vi "Read PIDs from Config.vi"(8 "error in (no error)":errorcluster, 10 "keys":string[](array[string]), 11 "Settings":variant) -> (0 "error out":errorcluster, 2 "Array":T1[](array[typedef]), 3 "Settings out":variant)   [LabVIEW 2019, in "DriveOld.lvlib" / "Drive.lvclass"]
doc: "This VI reads the PIDF values from the configuration file and returns an array of the PIDF's requested from the specific variant."
uses:
  Drive.lvclass
  <vilib>/Rock Robotics/WPI/ThirdParty/Phoenix-LabVIEW/Motor Controller/Controls/CTRE_Phoenix_MotorControl_SlotStructure.ctl
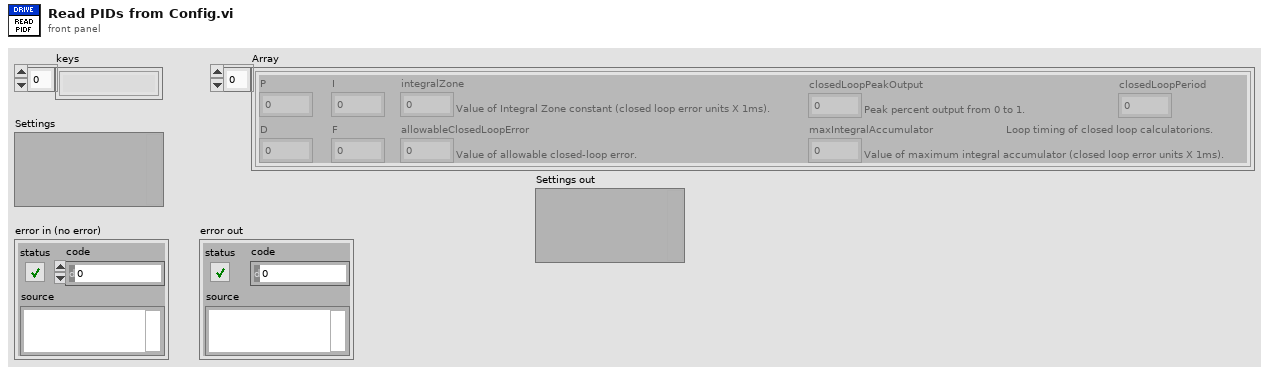
[diagram p1: front panel]
types:
  T1 = typedef "CTRE_Phoenix_MotorControl_SlotStructure.ctl" = cluster{"P":dbl, "I":dbl, "D":dbl, "F":dbl, "integralZone":dbl, "allowableClosedLoopError":i32, "maxIntegralAccumulator":dbl, "closedLoopPeakOutput":dbl, "closedLoopPeriod":i32}
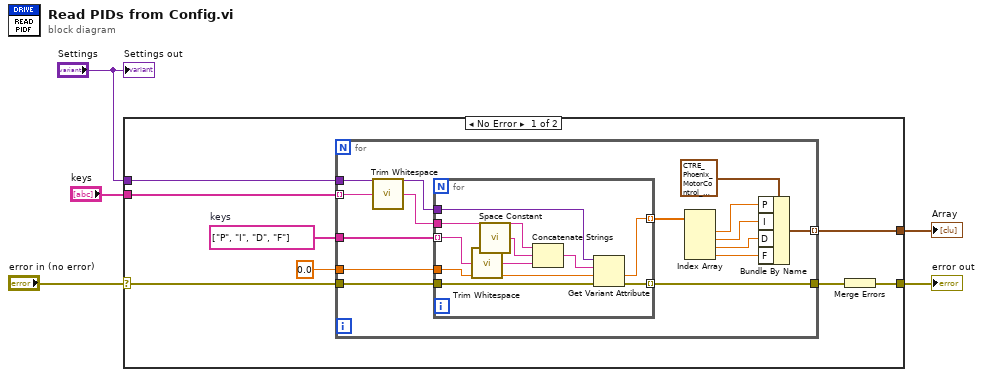
[diagram p0: block diagram]
diagram:
  n1 = case shown="No Error" "error in (no error)" {
    selector: "error in (no error)" -> [w10 w38]
    tunnel: [w12 w38] -> w5
    tunnel: "keys" -> [w9 _]
    tunnel: "Settings" -> [w8 _]
    tunnel: [w6 _] -> w1
    frame No Error {
      w7 = string[] ["P", "I", "D", "F"]  # keys
      n2 = for {
        tunnel: w8 -> [w27]
        tunnel: w9 -> [w22] mode=indexing
        tunnel: w10 -> [w26]
        tunnel: [w25] -> w11
        tunnel: 0.0 -> [w24]
        tunnel: w7 -> [w23]
        tunnel: [w15] -> w6 mode=indexing
        n3 = call <vilib>:"Trim Whitespace.vi"("string"=w22) -> ("trimmed string"=w21:string)  [unwired: 1 in]
        n4 = for {
          tunnel: [w37] -> w14 mode=indexing
          tunnel: w27 -> [w36]
          tunnel: w26 -> [w33]
          tunnel: [w32] -> w25 mode=indexing
          tunnel: w24 -> [w31]
          tunnel: w23 -> [w30] mode=indexing
          tunnel: w21 -> [w28]
          n5 = call <vilib>:"Trim Whitespace.vi"("string"=w30) -> ("trimmed string"=w29:string)  [unwired: 1 in]
          n6 = call <vilib>:"Space Constant.vi"() -> ("String"=w35:string)
          n7 = Concatenate Strings(w28, w35, w29) -> (w34:string)
          n8 = Get Variant Attribute(Variant=w36, name=w34, default value (empty Variant)=w31, error in=w33) -> (value=w37:dbl, error out=w32:errorcluster)  [unwired: 2 out]
        }
        n9 = Index Array(array=w14) -> (element #1=w20:dbl, element #2=w19:dbl, element #3=w18:dbl, element #4=w17:dbl)  [unwired: 4 in]
        n10 = Bundle By Name(cluster=T1 {"P"=0.0, "I"=0.0, "D"=0.0, "F"=0.0, "integralZone"=0.0, "allowableClosedLoopError"=0, "maxIntegralAccumulator"=0.0, "closedLoopPeakOutput"=1.0, "closedLoopPeriod"=1} ("Elevator Wrist PID"), "P"=w20, "I"=w19, "D"=w18, "F"=w17) -> (w15:T1)
      }
      n11 = Merge Errors(w11) -> (w12:errorcluster)
    }
    frame Error {
    }
  }
  "error out" <- w5
  "Array" <- w1
  "Settings out" <- "Settings"
